vi "_PC_D999 config_param.vi"(7 "Enum":enum8{"None", "Write", "Read"}(ring), 8 "error in (no error)":errorcluster, 11 "Refnum cluster in":T2) -> (0 "error out":errorcluster, 2 "data cluster output":T1, 3 "Refnum cluster out":T2)   [LabVIEW 2018]
uses:
  Constant/AccessFolderName.ctl
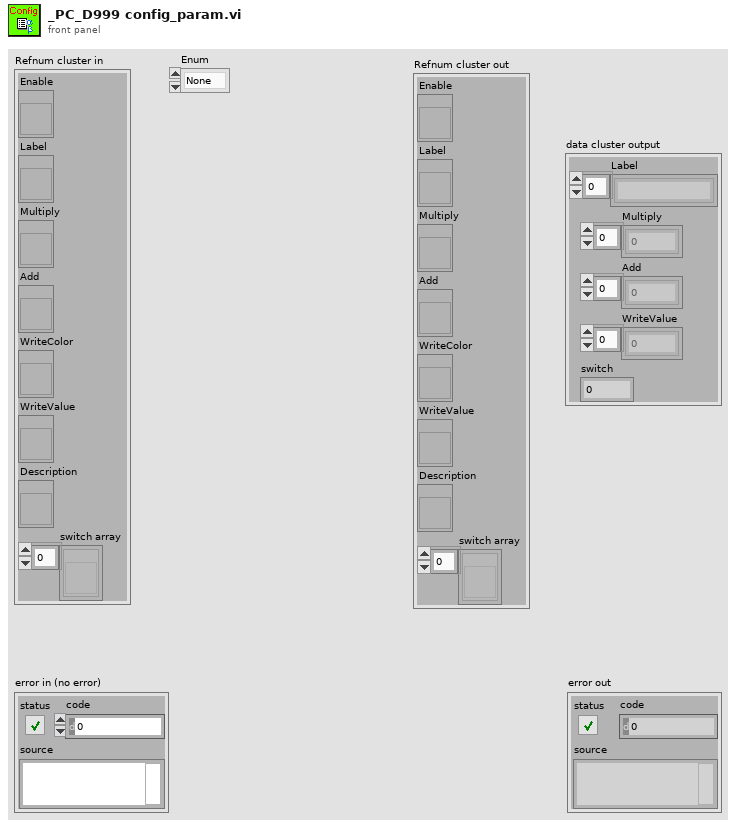
[diagram p1: front panel]
types:
  T1 = cluster{"Label":string[], "Multiply":dbl[], "Add":dbl[], "WriteValue":i16[], "switch":u32}
  T2 = cluster{"Enable":refnum<vi>, "Label":refnum<vi>, "Multiply":refnum<vi>, "Add":refnum<vi>, "WriteColor":refnum<vi>, "WriteValue":refnum<vi>, "Description":refnum<vi>, "switch array":refnum<vi>[]}
  T3 = typedef "AccessFolderName.ctl" = enum16{"None", "system_log", "ui_log", "msdata", "method", "d999_param"}
  T4 = enum16{"open", "replace", "create", "open or create", "replace or create", "replace or create with confirmation"}
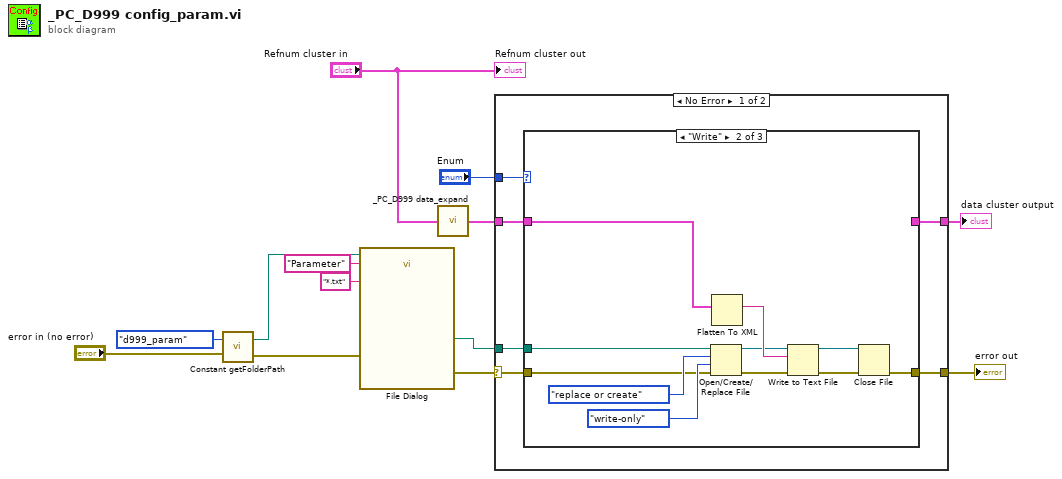
[diagram p0: block diagram]
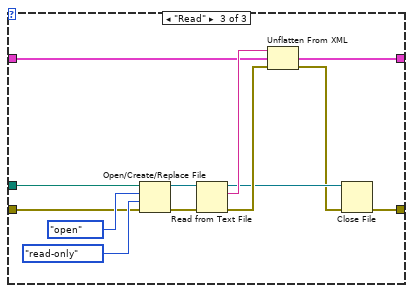
[diagram p3: hidden frame]
diagram:
  n1 = call "Constant getFolderPath.vi"("error in (no error)"="error in (no error)", "folder name"=AccessFolderName."d999_param") -> ("error out"=w4:errorcluster, "folder path"=w3:path)
  n2 = call "File Dialog"("start path"=w3, "default name"="Parameter", "error in"=w4, "pattern (all files)"="*.txt") -> ("selected path"=w9:path, "error out"=w7:errorcluster)  [unwired: 8 in, 2 out]
  n3 = call "_PC_D999 data_expand.vi"("Refnum cluster in"="Refnum cluster in") -> ("data cluster output"=w10:T1)
  n4 = case shown="No Error" w7 {
    selector: w7 -> [w15 w45]
    tunnel: "Enum" -> [w19 _]
    tunnel: w10 -> [w18 _]
    tunnel: w9 -> [w17 _]
    tunnel: [w16 w45] -> w8
    tunnel: [w14 _] -> w1
    frame No Error {
      n5 = case shown="\"Write\"" w19 {
        tunnel: w17 -> [_ w27 w39]
        tunnel: [w20 w21 w34] -> w16
        tunnel: w15 -> [w20 w26 w38]
        tunnel: w18 -> [_ w30 w42]
        tunnel: [_ _ w33] -> w14
        frame "None", Default {
        }
        frame "Write" {
          n6 = Open/Create/Replace File(file path (use dialog)=w27, error in=w26, operation (0:open)=T4."replace or create", access (0:read/write)=enum16{"read/write", "read-only", "write-only"}."write-only") -> (refnum out=w25:refnum<file>, error out=w24:errorcluster)  [unwired: 2 in, 1 out]
          n7 = Flatten To XML(anything=w30) -> (xml string=w31:string)
          n8 = Write to Text File(file (use dialog)=w25, text=w31, error in=w24) -> (refnum out=w23:refnum<file>, error out=w22:errorcluster)  [unwired: 1 in, 1 out]
          n9 = Close File(refnum=w23, error in=w22) -> (error out=w21:errorcluster)  [unwired: 1 out]
        }
        frame "Read" {
          n10 = Open/Create/Replace File(file path (use dialog)=w39, error in=w38, operation (0:open)=T4."open", access (0:read/write)=enum16{"read/write", "read-only", "write-only"}."read-only") -> (refnum out=w37:refnum<file>, error out=w36:errorcluster)  [unwired: 2 in, 1 out]
          n11 = Read from Text File(file (use dialog)=w37, error in=w36) -> (refnum out=w35:refnum<file>, text=w44:string, error out=w43:errorcluster)  [unwired: 2 in, 1 out]
          n12 = Unflatten From XML(xml string=w44, type=w42, error in (no error)=w43) -> (value=w33:T1, error out=w32:errorcluster)
          n13 = Close File(refnum=w35, error in=w32) -> (error out=w34:errorcluster)  [unwired: 1 out]
        }
      }
    }
    frame Error {
    }
  }
  "error out" <- w8
  "data cluster output" <- w1
  "Refnum cluster out" <- "Refnum cluster in"
